vi "Start Capturing.vi"(7 "DO Channel":u8=7, 8 "Error In":errorcluster, 9 "Start Capture":bool, 10 "Half capture time":u32=750, 11 "LINX Resource":T1) -> (0 "Error Out":errorcluster, 3 "LINX Resource 2":T1)   [LabVIEW 2014]
uses:
  <vilib>/MakerHub/LINX/Private/Type Defs/LINX Ref.ctl
  <vilib>/MakerHub/LINX/Private/Type Defs/Platform.ctl
  <vilib>/MakerHub/LINX/Private/Type Defs/Interface.ctl
  <vilib>/MakerHub/LINX/Private/Device/Type Defs/LINX Device Config.ctl
  <vilib>/MakerHub/LINX/Private/Device/Type Defs/TCP Config.ctl
  <vilib>/MakerHub/LINX/Private/Device/Type Defs/Channels.ctl
  <vilib>/MakerHub/LINX/Public/Peripherals/Digital/Digital Write 1 Chan.vi
  <vilib>/MakerHub/LINX/Public/Peripherals/Digital/Digital Write N Chans.vi
  <vilib>/MakerHub/LINX/Private/Local IO/LinxDigitalWrite.vi
  <vilib>/MakerHub/LINX/Public/Utilities/Check Channel.vi
  <vilib>/MakerHub/LINX/Private/Local IO/Handle Errors.vi
  FGV/Camer Control Variables.vi
  <vilib>/MakerHub/LINX/Private/Utilties/Generate Error.vi
  <vilib>/MakerHub/LINX/LMH-LINX.lvlib
  <vilib>/MakerHub/LINX/Private/Device/Device.lvlib
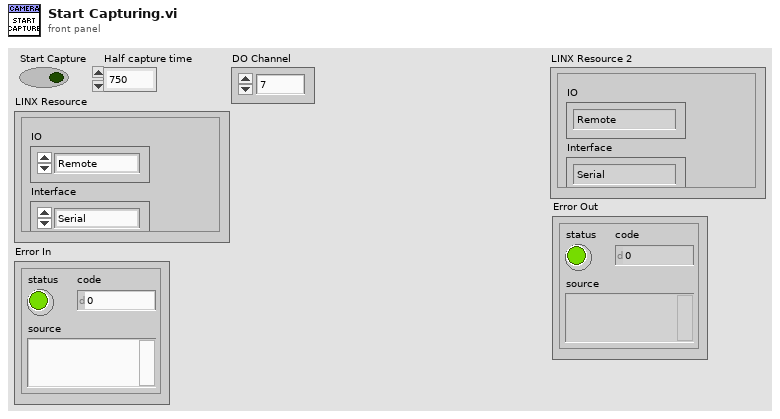
[diagram p1: front panel]
types:
  T1 = typedef "LMH-LINX.lvlib/LINX Ref.ctl" = cluster{"IO":T2, "Interface":T3, "LINX Device Config":T4}
  T2 = typedef "LMH-LINX.lvlib/Platform.ctl" = enum16{"Remote", "Local"}
  T3 = typedef "LMH-LINX.lvlib/Interface.ctl" = enum16{"Serial", "TCP"}
  T4 = typedef "LMH-LINX.lvlib/Device.lvlib/LINX Device Config.ctl" = cluster{"Interface":T3, "COM Port":refnum<visa-resource-name>, "TCP Configuration":T5, "Device Family":u8, "Device ID":u8, "Device Name":string, "TCP Ref":refnum<k5>, "Channels":T6}
  T5 = typedef "LMH-LINX.lvlib/Device.lvlib/TCP Config.ctl" = cluster{"IP Address":string, "Port":u16}
  T6 = typedef "LMH-LINX.lvlib/Channels.ctl" = cluster{"DI":u8[], "DO":u8[], "AI":u8[], "AO":u8[], "PWM":u8[], "QE":u8[], "UART":u8[], "I2C 2":u8[], "SPI":u8[], "CAN":u8[], "Servo":u8[], "AI Ref (V)":dbl, "AI Resolution (Bits)":u8, "AO Ref (V)":dbl, "AO Resolution (Bits)":u8}
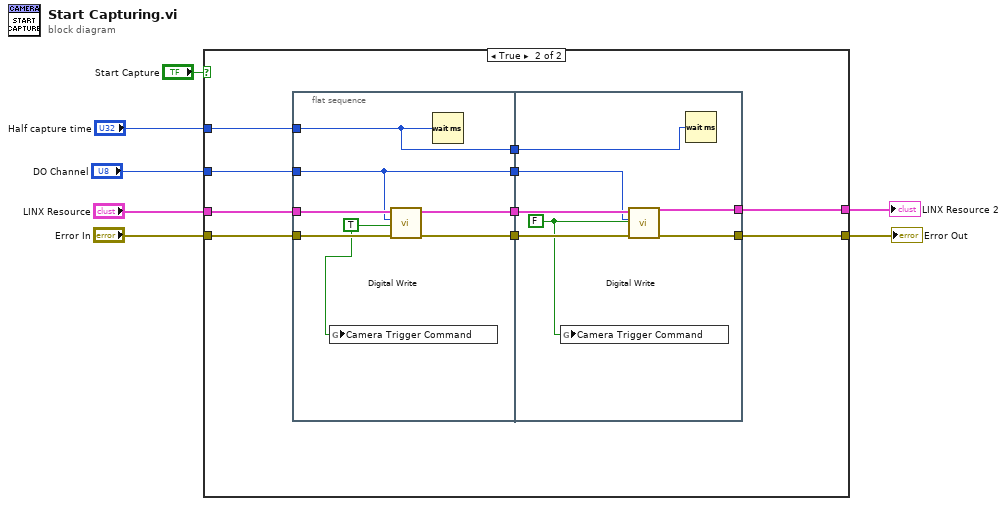
[diagram p0: block diagram]
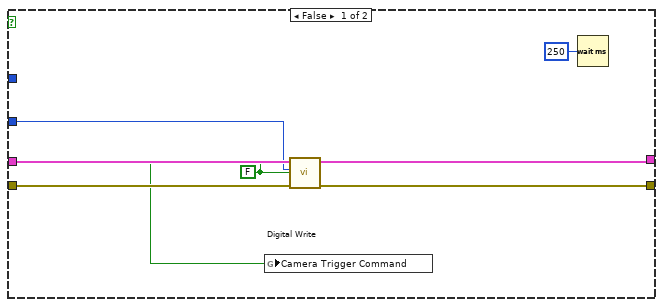
[diagram p2: hidden frame]
diagram:
  n1 = case shown="True" "Start Capture" {
    tunnel: "LINX Resource" -> [w10 w24]
    tunnel: "Error In" -> [w13 w23]
    tunnel: "DO Channel" -> [w9 w22]
    tunnel: "Half capture time" -> [_ w18]
    tunnel: [w12 w16] -> w2
    tunnel: [w11 w15] -> w1
    frame False {
      w8 = FALSE ("Output Value")
      n2 = global write "Camer Control Variables.vi" "Camera Trigger Command"(w8) -> ()
      n3 = call-poly <vilib>:"Digital Write.vi"("Error In"=w13, "Output Value"=w8, "DO Channel"=w9, "LINX Resource"=w10) -> ("Error Out"=w12:errorcluster, "LINX Resource"=w11:T1)  [unwired: 6 in]
      n4 = Wait (ms)(milliseconds to wait=u32 250) -> ()  [unwired: 1 out]
    }
    frame True {
      n5 = flat-sequence {
        tunnel: w24 -> [w31]
        tunnel: w23 -> [w30]
        tunnel: w22 -> [w27]
        tunnel: [w29] -> w21
        tunnel: [w28] -> w20
        tunnel: [w27] -> w19
        tunnel: w18 -> [w26]
        tunnel: [w26] -> w17
        tunnel: w21 -> [w38]
        tunnel: w20 -> [w37]
        tunnel: w19 -> [w36]
        tunnel: w17 -> [w35]
        tunnel: [w34] -> w16
        tunnel: [w33] -> w15
        frame #0 {
          w25 = TRUE ("Output Value")
          n6 = global write "Camer Control Variables.vi" "Camera Trigger Command"(w25) -> ()
          n7 = call-poly <vilib>:"Digital Write.vi"("Error In"=w30, "Output Value"=w25, "DO Channel"=w27, "LINX Resource"=w31) -> ("Error Out"=w28:errorcluster, "LINX Resource"=w29:T1)  [unwired: 6 in]
          n8 = Wait (ms)(milliseconds to wait=w26) -> ()  [unwired: 1 out]
        }
        frame #1 {
          w32 = FALSE ("Output Value")
          n9 = global write "Camer Control Variables.vi" "Camera Trigger Command"(w32) -> ()
          n10 = call-poly <vilib>:"Digital Write.vi"("Error In"=w37, "Output Value"=w32, "DO Channel"=w36, "LINX Resource"=w38) -> ("Error Out"=w34:errorcluster, "LINX Resource"=w33:T1)  [unwired: 6 in]
          n11 = Wait (ms)(milliseconds to wait=w35) -> ()  [unwired: 1 out]
        }
      }
    }
  }
  "LINX Resource 2" <- w1
  "Error Out" <- w2
